vi "五子棋_電腦對戰V2.vi"() -> ()   [LabVIEW 2019, in "五子棋.lvlib"]
uses:
  Status.ctl
  SetPiece.ctl
  Piece.ctl
  <vilib>/numeric/Random Number (Range) U64.vi
  1e88ba00-7128-4acd-b617-a9aca016128f.vi
  <vilib>/numeric/sub_Random U32.vi
panel:
  out "Info":string
  out "狀態":string
  out "黑子":T1[][](array[typedef])
  out "白子":T2[][](array[typedef])
  out "Score":i32[][](array[numeric])
  # "五子棋電腦對戰版"
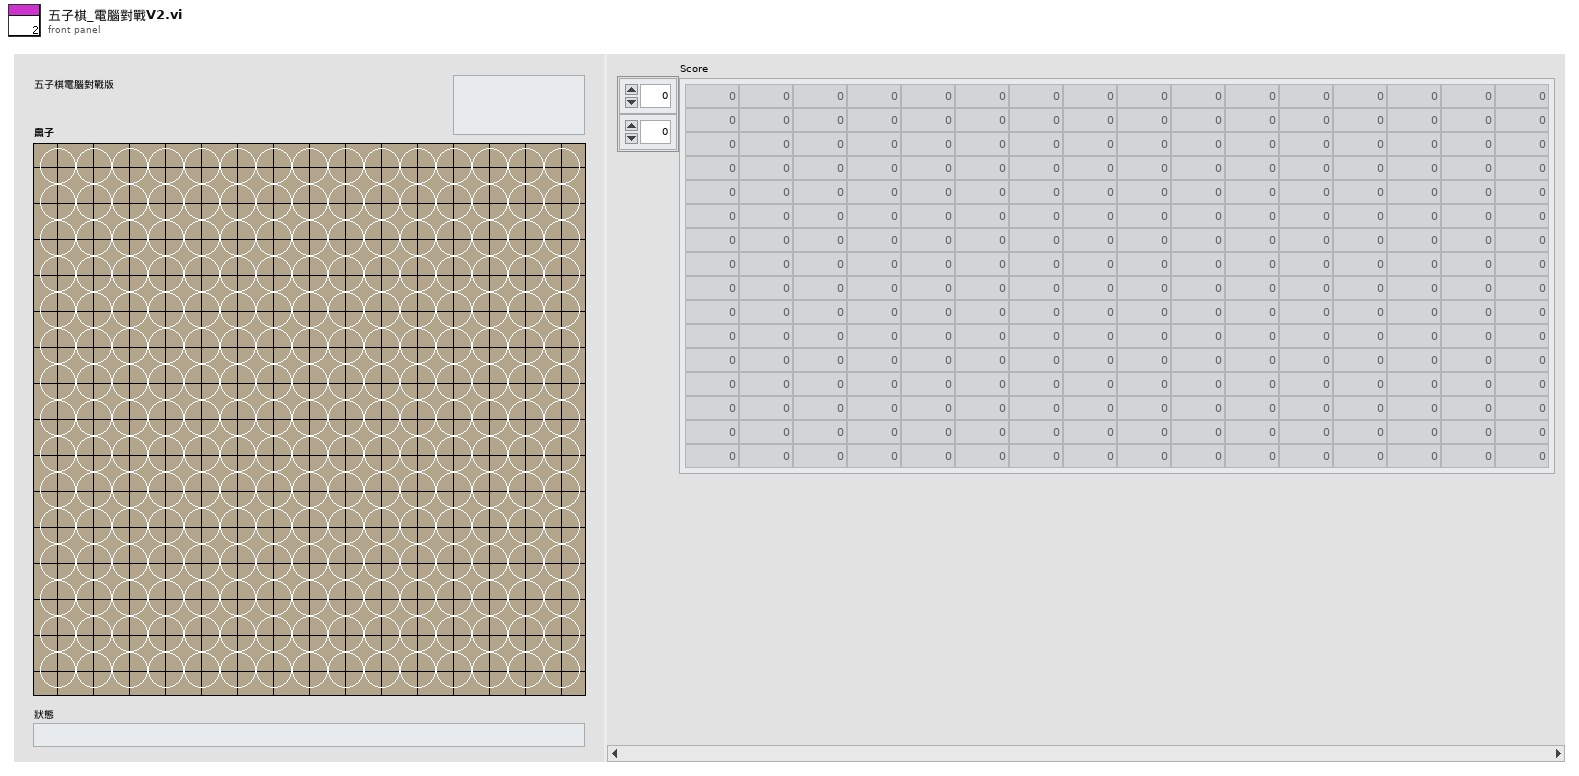
[diagram p1: front panel]
types:
  T1 = typedef "五子棋.lvlib/黑子.ctl" = bool
  T2 = typedef "五子棋.lvlib/白子.ctl" = bool
  T3 = typedef "五子棋.lvlib/Piece.ctl" = enum16{"None", "Black", "White"}
  T4 = typedef "五子棋.lvlib/SetPiece.ctl" = cluster{"Row":i32, "Col":i32}
  T5 = typedef "五子棋.lvlib/Status.ctl" = enum16{"Idle", "Initialize", "Set Piece", "Check Win", "Computer Play"}
  T6 = typedef "LVPositionTypeDef.ctl" = cluster{"Left":i32, "Top":i32}
  T7 = typedef "LVBoundsTypeDef.ctl" = cluster{"Width":u32, "Height":u32}
  T8 = cluster{"Number of Columns":u32, "Number of Rows":u32}
  T9 = typedef "LVPoint32TypeDef.ctl" = cluster{"Horizontal":i32, "Vertical":i32}
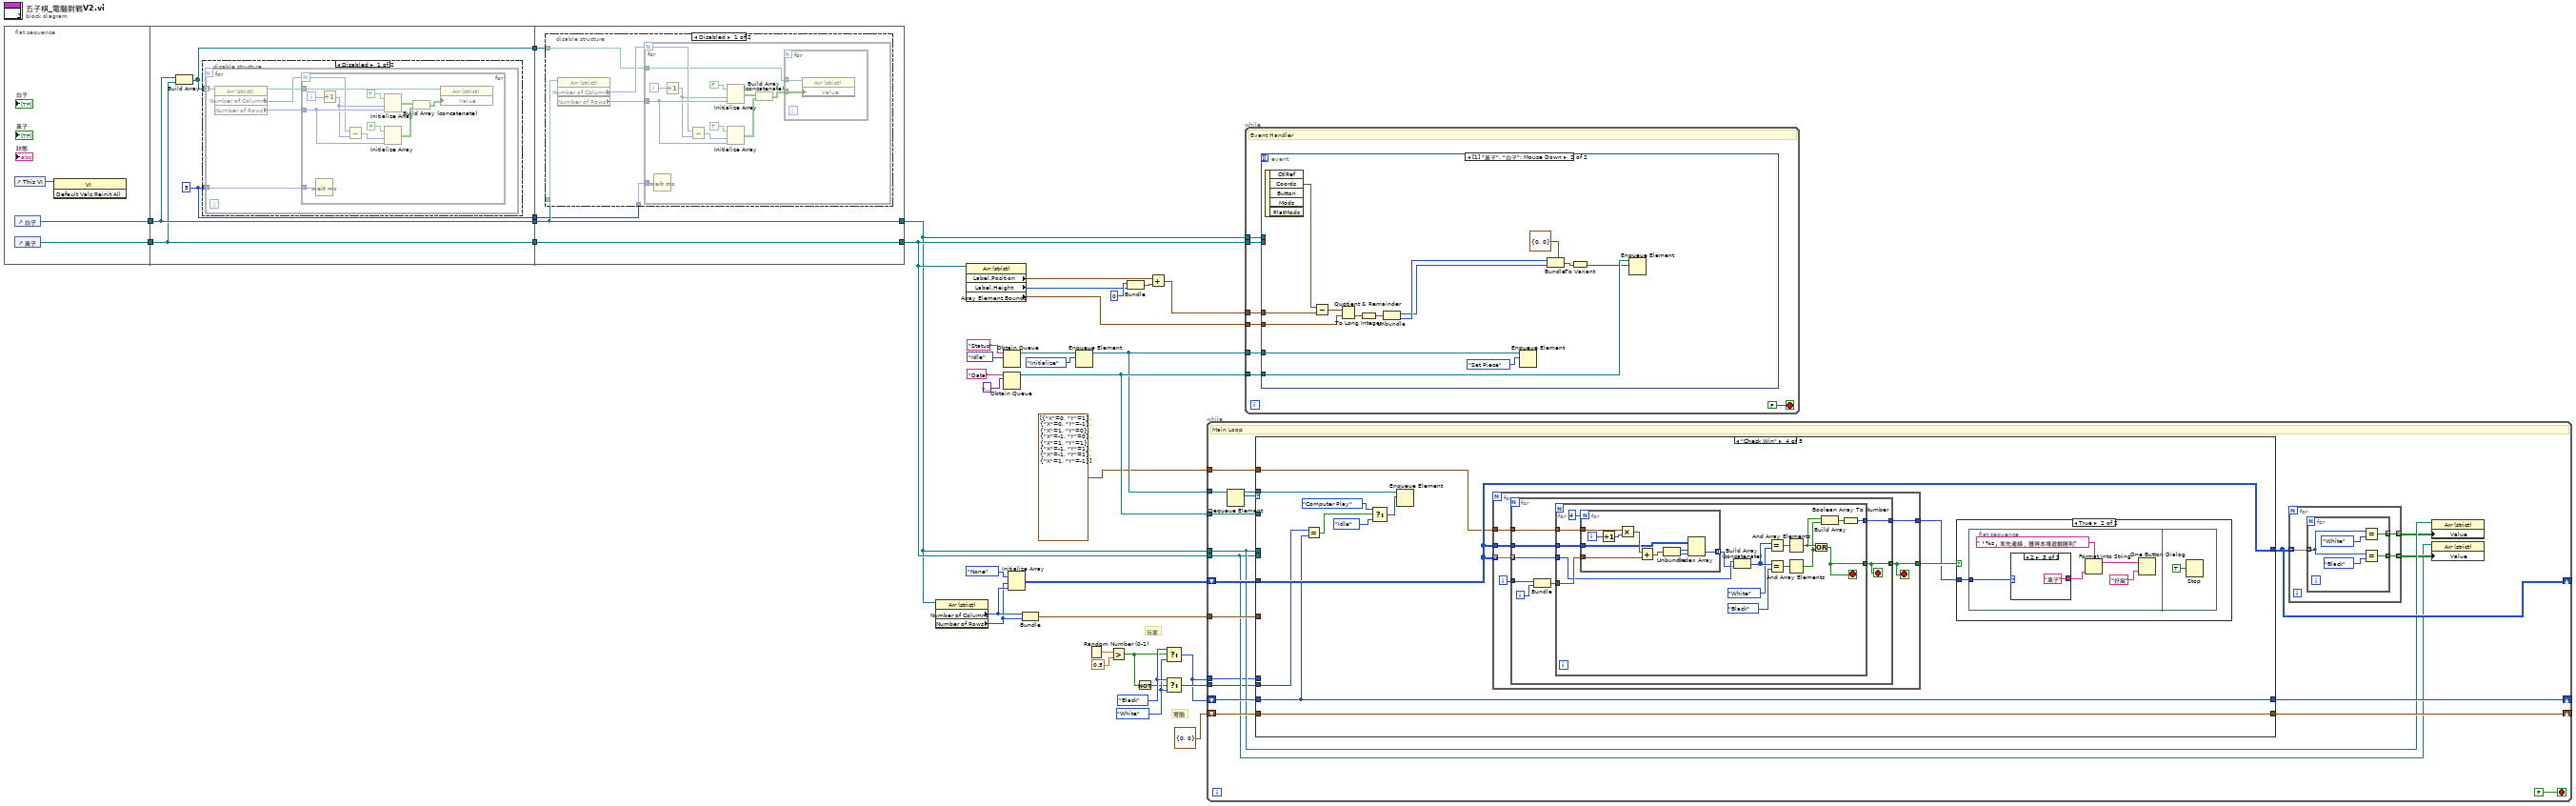
[diagram p0: block diagram]
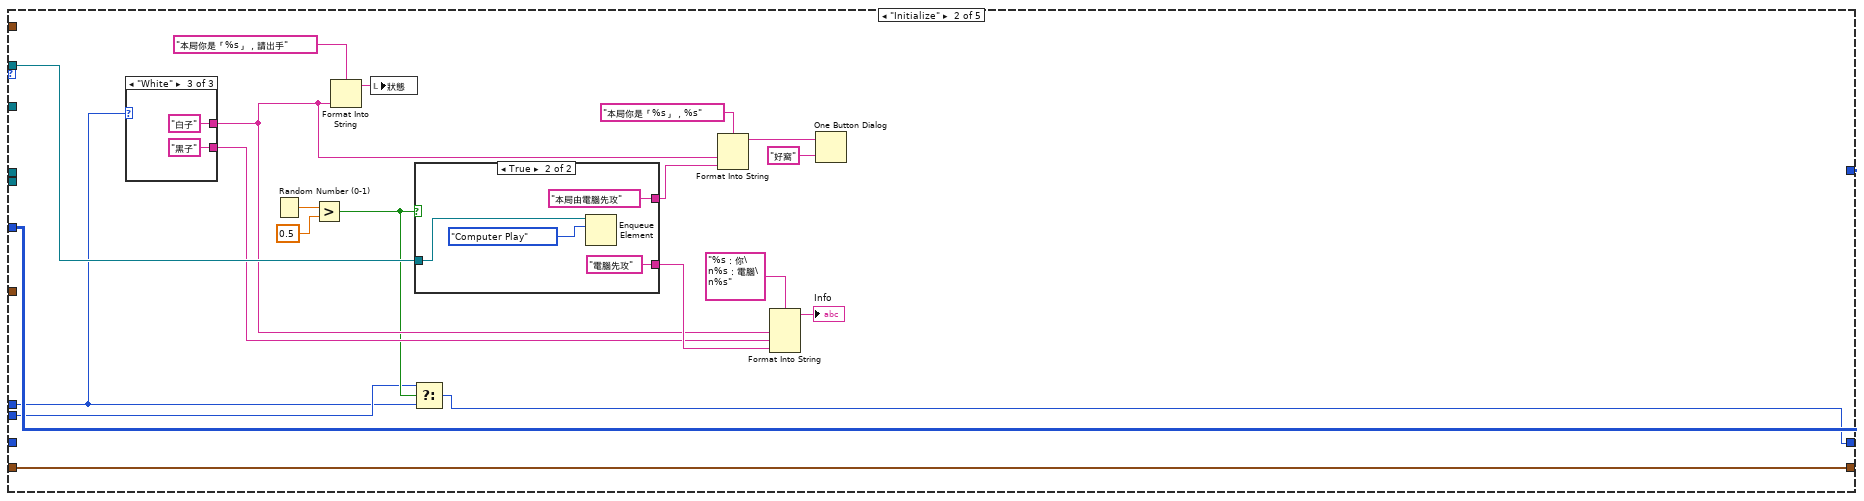
[diagram p5: hidden frame]
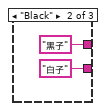
[diagram p7: hidden frame]
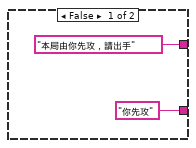
[diagram p8: hidden frame]
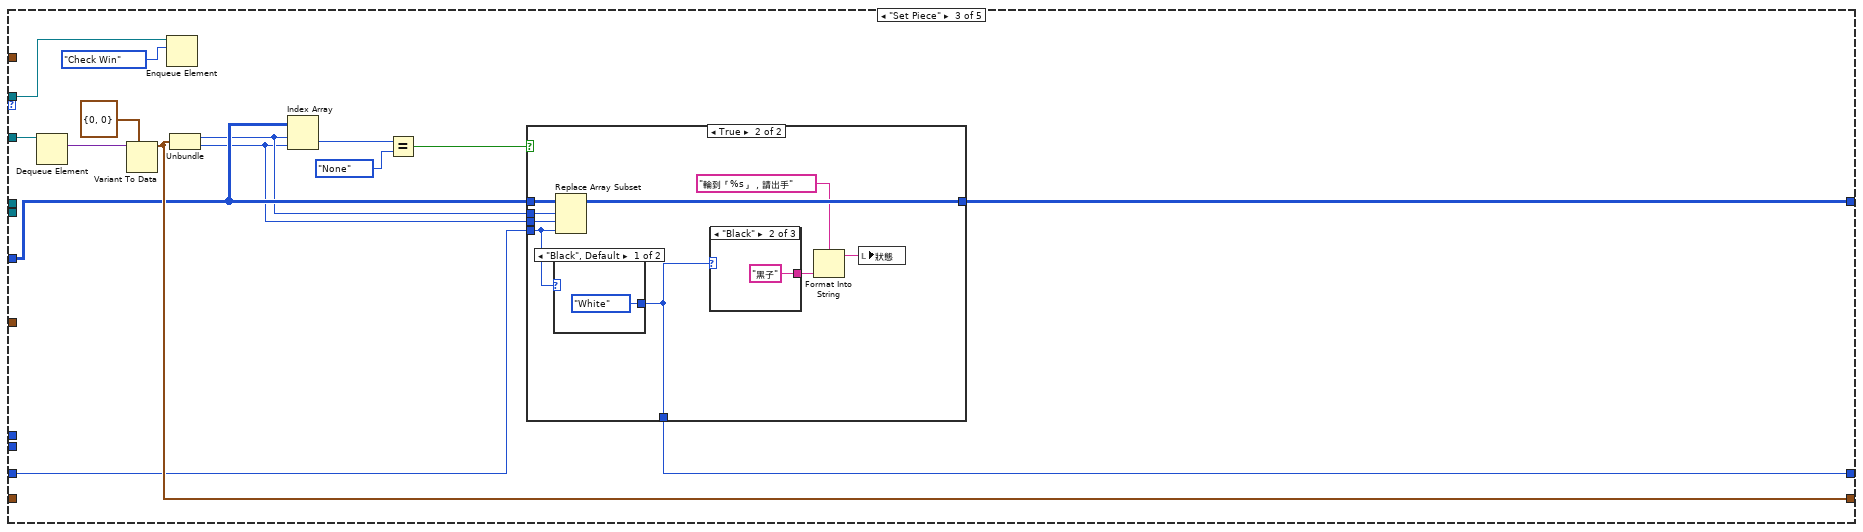
[diagram p9: hidden frame]
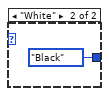
[diagram p11: hidden frame]
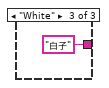
[diagram p13: hidden frame]
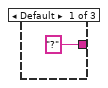
[diagram p15: hidden frame]
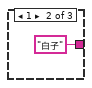
[diagram p16: hidden frame]
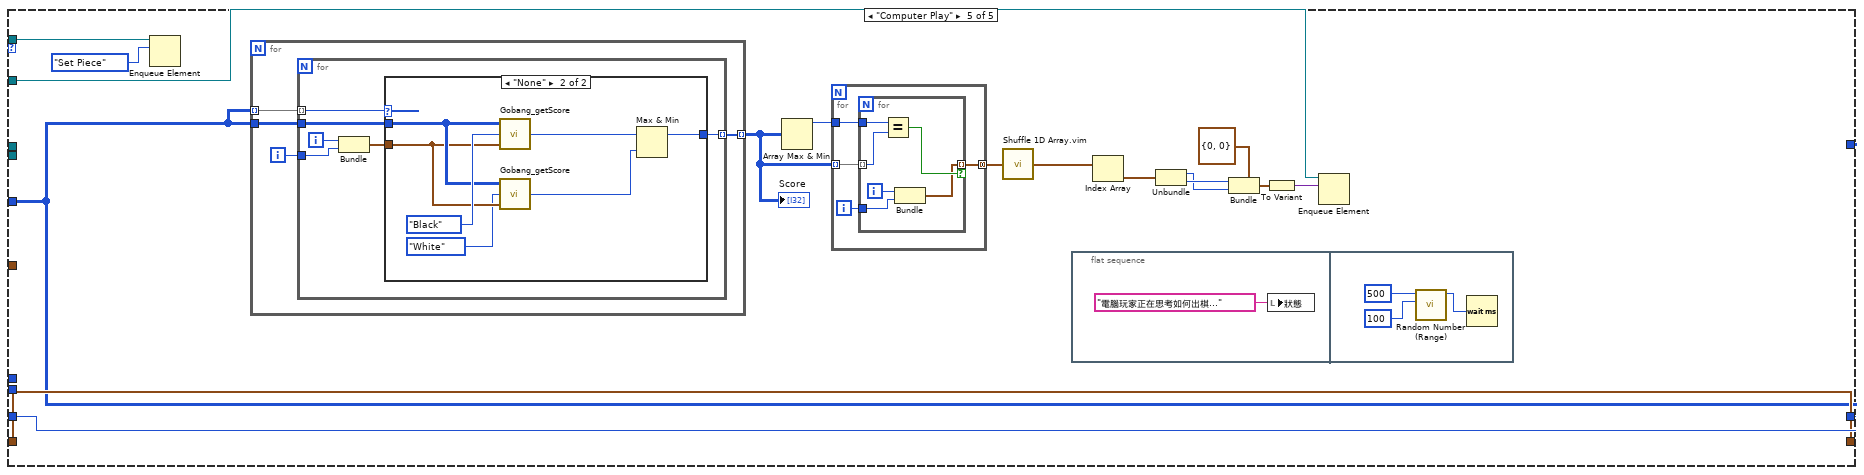
[diagram p17: hidden frame]
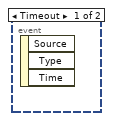
[diagram p19: hidden frame]
diagram:
  w7 = Piece."White" ("new element/subarray")
  w8 = Piece."Black" ("new element/subarray")
  # "電腦"
  # "玩家"
  n1 = flat-sequence {
    tunnel: [w39] -> w21
    tunnel: [w38] -> w20
    tunnel: w21 -> [w43]
    tunnel: w20 -> [w44]
    tunnel: [w43] -> w19
    tunnel: [w44] -> w18
    tunnel: [w42] -> w17
    tunnel: [w41] -> w13
    tunnel: [w66] -> w15
    tunnel: [w67] -> w32
    tunnel: w19 -> [w67]
    tunnel: w18 -> [w66]
    tunnel: w17 -> [w65]
    tunnel: w13 -> [w64]
    frame #0 {
      n2 = control-ref of="This VI"() -> (w40:refnum<vi>)
      n3 = control-ref of="白子"() -> (w38:refnum<vi>)
      n4 = control-ref of="黑子"() -> (w39:refnum<vi>)
      n5 = invoke class="VI" method="Default Vals.Reinit All"(reference=w40) -> ()  [unwired: 2 in, 3 out]
    }
    frame #1 {
      w41 = u32 5 ("milliseconds to wait")
      n6 = Build Array(w44, w43) -> (w42:refnum<vi>[])
      n7 = disable-structure shown="Disabled" {
        disable-tunnel: w42 -> [w46 _]
        disable-tunnel: w41 -> [w45 _]
        frame Disabled {
          n8 = for {
            tunnel: w46 -> [w51] mode=indexing
            tunnel: w45 -> [w47]
            n9 = property class="Arr (strict)"(reference=w51) -> (reference out=w48:refnum<vi>, "Number of Columns"=w50:u32, "Number of Rows"=w49:u32)  [unwired: 1 in, 1 out]
            n10 = for {
              N: w50 -> [w59]
              tunnel: w49 -> [w60]
              tunnel: w48 -> [w54]
              tunnel: w47 -> [w52]
              i -> [w62]
              n11 = Wait (ms)(milliseconds to wait=w52) -> ()  [unwired: 1 out]
              n12 = Increment(x=w62) -> (x+1=w58:i32)
              n13 = Subtract(x=w59, y=w58) -> (x-y=w57:i32)
              n14 = Initialize Array(TRUE, w58, w60) -> (w56:bool[][])
              n15 = Initialize Array(FALSE, w57, w60) -> (w55:bool[][])
              n16 = Build Array (concatenate)(w56, w55) -> (w53:bool[][])
              n17 = property class="Arr (strict)"(reference=w54, "Value"=w53) -> ()  [unwired: 1 in, 2 out]
            }
          }
        }
        frame Enabled {
        }
      }
    }
    frame #2 {
      n18 = disable-structure shown="Disabled" {
        disable-tunnel: w66 -> [w70 _]
        disable-tunnel: w65 -> [w69 _]
        disable-tunnel: w64 -> [w68 _]
        frame Disabled {
          n19 = property class="Arr (strict)"(reference=w70) -> ("Number of Columns"=w72:u32, "Number of Rows"=w71:u32)  [unwired: 1 in, 2 out]
          n20 = for {
            N: w72 -> [w80]
            tunnel: w71 -> [w81]
            tunnel: w69 -> [w74]
            tunnel: w68 -> [w73]
            i -> [w83]
            n21 = Wait (ms)(milliseconds to wait=w73) -> ()  [unwired: 1 out]
            n22 = Increment(x=w83) -> (x+1=w79:i32)
            n23 = Subtract(x=w80, y=w79) -> (x-y=w78:i32)
            n24 = Initialize Array(FALSE, w79, w81) -> (w77:bool[][])
            n25 = Initialize Array(TRUE, w78, w81) -> (w76:bool[][])
            n26 = Build Array (concatenate)(w77, w76) -> (w75:bool[][])
            n27 = for {
              tunnel: w74 -> [w86] mode=indexing
              tunnel: w75 -> [w85]
              n28 = property class="Arr (strict)"(reference=w86, "Value"=w85) -> ()  [unwired: 1 in, 2 out]
            }
          }
        }
        frame Enabled {
        }
      }
    }
  }
  n29 = property class="Arr (strict)"(reference=w15) -> ("Number of Columns"=w11:u32, "Number of Rows"=w10:u32)  [unwired: 1 in, 2 out]
  n30 = property class="Arr (strict)"(reference=w32) -> ("Label.Position"=w31:T6, "Label.Height"=w27:u32, "Array Element.Bounds"=w26:T7)  [unwired: 1 in, 2 out]
  n31 = Obtain Queue(name (unnamed)="Status", element data type=Status."Idle" ("Status")) -> (queue out=w23:refnum<queue>)  [unwired: 3 in, 2 out]
  n32 = Obtain Queue(name (unnamed)="Data", element data type=variant) -> (queue out=w33:refnum<queue>)  [unwired: 3 in, 2 out]
  n33 = Initialize Array(Piece."None", w10, w11) -> (w9:T3[][])
  n34 = Bundle("Number of Columns"=w11, "Number of Rows"=w10) -> (w3:T8)  [unwired: 1 in]
  n35 = Enqueue Element(queue=w23, element=Status."Initialize" ("Status")) -> (queue out=w14:refnum<queue>)  [unwired: 2 in, 2 out]
  n36 = Random Number (0-1)() -> (number: 0 to 1=w25:dbl)
  n37 = Greater?(x=w25, y=0.5) -> (0:w6:bool)
  n38 = Bundle(0, "Label.Height"=w27) -> (w30:cluster{i32, "Label.Height":u32})  [unwired: 1 in]
  n39 = Not(x=w6) -> (.not. x?=w5:bool)
  n40 = Add(x=w31, y=w30) -> (x+y=w29:cluster{i32, u32})
  n41 = Select(t=w8, s=w6, f=w7) -> (s? t:f=w1:T3)
  n42 = Select(t=w8, s=w5, f=w7) -> (s? t:f=w4:T3)
  n43 = while {
    tunnel: w14 -> [w104]
    tunnel: w33 -> [w100]
    tunnel: w32 -> [w90]
    tunnel: w15 -> [w93]
    shift-right: [w99] -> _
    shift-left: w1 -> [w98]
    shift-right: [w97] -> _
    shift-left: T4 {"Row"=0, "Col"=0} -> [w96]
    tunnel: w3 -> [w95]
    shift-right: [w105] -> _
    shift-left: w9 -> [w94]
    tunnel: w1 -> [w89]
    tunnel: w4 -> [w88]
    tunnel: cluster{"X":i32, "Y":i32}[] [{"X"=0, "Y"=1}, {"X"=0, "Y"=-1}, {"X"=1, "Y"=0}, {"X"=-1, "Y"=0}, {"X"=1, "Y"=1}, {"X"=-1, "Y"=1}, {"X"=-1, "Y"=1}, {"X"=1, "Y"=-1}] -> [w87]
    stop <- FALSE stop-if-true
    # "Main Loop"
    n44 = Dequeue Element(queue=w104) -> (queue out=w101:refnum<queue>, element=w103:T5)  [unwired: 2 in, 2 out]
    n45 = case shown="\"Check Win\"" w103 {
      tunnel: w90 -> [_ _ _ _ _]
      tunnel: w93 -> [_ _ _ _ _]
      tunnel: w101 -> [_ w125 w152 w180 w246]
      tunnel: w100 -> [_ _ w150 _ w240]
      tunnel: [w108 w109 w139 w171 w245] -> w99
      tunnel: w98 -> [w108 _ w146 w171 w245]
      tunnel: [w107 w126 w148 w174 w243] -> w97
      tunnel: w96 -> [w107 w126 _ w174 w243]
      tunnel: w95 -> [_ _ _ _ _]
      tunnel: w94 -> [w106 w115 w145 w173 w242]
      tunnel: [w106 w115 w147 w173 w242] -> w105
      tunnel: w89 -> [_ w110 _ _ _]
      tunnel: w88 -> [_ w111 _ w170 _]
      tunnel: w87 -> [_ _ _ w169 _]
      frame "Idle", Default {
      }
      frame "Initialize" {
        n46 = case shown="\"White\"" w110 {
          tunnel: [_ "黑子" "白子"] -> w114
          tunnel: [_ "白子" "黑子"] -> w113
          frame Default {
          }
          frame "Black" {
          }
          frame "White" {
          }
        }
        n47 = Random Number (0-1)() -> (number: 0 to 1=w123:dbl)
        n48 = Greater?(x=w123, y=0.5) -> (0:w112:bool)
        n49 = Format Into String(format string="本局你是「%s」，請出手", w114) -> (resulting string=w127:string)  [unwired: 2 in, 1 out]
        n50 = local write "狀態"(w127) -> ()
        n51 = Select(t=w111, s=w112, f=w110) -> (s? t:f=w109:T3)
        n52 = case shown="True" w112 {
          tunnel: w125 -> [_ w136]
          tunnel: ["本局由你先攻，請出手" ("format string") "本局由電腦先攻" ("format string")] -> w121
          tunnel: ["你先攻" ("format string") "電腦先攻" ("format string")] -> w117
          frame False {
          }
          frame True {
            n53 = Enqueue Element(queue=w136, element=Status."Computer Play" ("Status")) -> ()  [unwired: 2 in, 3 out]
          }
        }
        n54 = Format Into String(format string="本局你是「%s」，%s", w114, w121) -> (resulting string=w120:string)  [unwired: 2 in, 1 out]
        n55 = Format Into String(format string="%s：你\n%s：電腦\n%s", w114, w113, w117) -> (resulting string=→"Info":string)  [unwired: 2 in, 1 out]
        n56 = One Button Dialog(message=w120, button name ("OK")="好窩") -> ()  [unwired: 1 out]
      }
      frame "Set Piece" {
        n57 = Dequeue Element(queue=w150) -> (element=w149:variant)  [unwired: 2 in, 3 out]
        n58 = Variant To Data(type=T4 {"Row"=0, "Col"=0}, Variant=w149) -> (data=w148:T4)  [unwired: 1 in, 1 out]
        n59 = Enqueue Element(queue=w152, element=Status."Check Win") -> ()  [unwired: 2 in, 3 out]
        n60 = Unbundle(w148) -> ("Row"=w144:i32, "Col"=w143:i32)
        n61 = Index Array(array=w145, index (row)=w144, index (col)=w143) -> (element=w142:T3)
        n62 = Equal?(x=w142, y=Piece."None") -> (x = y?=w140:bool)
        n63 = case shown="True" w140 {
          tunnel: [w155 w164] -> w147
          tunnel: w146 -> [w154 w158]
          tunnel: w145 -> [w155 w163]
          tunnel: w144 -> [_ w162]
          tunnel: w143 -> [_ w161]
          tunnel: [w154 w156] -> w139
          frame False {
          }
          frame True {
            n64 = case shown="\"Black\", Default" w158 {
              tunnel: [Piece."White" ("new element/subarray") Piece."Black" ("new element/subarray")] -> w156
              frame "Black", Default {
              }
              frame "White" {
              }
            }
            n65 = Replace Array Subset(array=w163, new element=w158, index (row)=w162, index (col)=w161) -> (w164:T3[][])
            n66 = case shown="\"Black\"" w156 {
              tunnel: [_ "黑子" "白子"] -> w160
              frame Default {
              }
              frame "Black" {
              }
              frame "White" {
              }
            }
            n67 = Format Into String(format string="輪到「%s」，請出手", w160) -> (resulting string=w159:string)  [unwired: 2 in, 1 out]
            n68 = local write "狀態"(w159) -> ()
          }
        }
      }
      frame "Check Win" {
        n69 = Equal?(x=w170, y=w171) -> (x = y?=w178:bool)
        n70 = Select(t=Status."Computer Play" ("element"), s=w178, f=Status."Idle" ("element")) -> (s? t:f=w177:T5)
        n71 = Enqueue Element(queue=w180, element=w177) -> ()  [unwired: 2 in, 3 out]
        n72 = for {
          tunnel: [w186] -> w179
          tunnel: w173 -> [w184] mode=indexing
          tunnel: w173 -> [w183]
          tunnel: [w182] -> w172
          tunnel: w169 -> [w181]
          i -> [w185]
          stop <- w186 stop-if-true
          n73 = for {
            tunnel: [w194] -> w186
            tunnel: w185 -> [w193]
            tunnel: w184 -> [w190] mode=indexing
            tunnel: w183 -> [w189]
            tunnel: [w188] -> w182
            tunnel: w181 -> [w187]
            i -> [w192]
            stop <- w194 stop-if-true
            n74 = Bundle(w193, w192) -> (w191:cluster{i32, i32})  [unwired: 1 in]
            n75 = for {
              tunnel: [w200] -> w194
              tunnel: w191 -> [w209]
              tunnel: w190 -> [w207]
              tunnel: w189 -> [w208]
              tunnel: [w196] -> w188
              tunnel: w187 -> [w195] mode=indexing
              stop <- w200 stop-if-true
              n76 = for {
                N: 4 -> [_]
                tunnel: w209 -> [w218]
                tunnel: w208 -> [w213]
                tunnel: [w212] -> w206 mode=indexing
                tunnel: w195 -> [w211]
                i -> [w217]
                n77 = Increment(x=w217) -> (x+1=w216:i32)
                n78 = Multiply(x=w211, y=w216) -> (x*y=w215:cluster{"X":i32, "Y":i32})
                n79 = Add(x=w215, y=w218) -> (x+y=w214:cluster{i32, i32})
                n80 = Unbundle(w214) -> (w220:i32, w219:i32)
                n81 = Index Array(array=w213, index (row)=w220, index (col)=w219) -> (element=w212:T3)
              }
              n82 = Build Array (concatenate)(w207, w206) -> (w202:T3[])
              n83 = Equal?(x=w202, y=Piece."White") -> (x = y?=w203:bool[])
              n84 = Equal?(x=w202, y=Piece."Black") -> (x = y?=w204:bool[])
              n85 = And Array Elements(Boolean array=w203) -> (logical AND=w199:bool)
              n86 = And Array Elements(Boolean array=w204) -> (logical AND=w198:bool)
              n87 = Or(x=w199, y=w198) -> (x .or. y?=w200:bool)
              n88 = Build Array(w199, w198) -> (w197:bool[])
              n89 = Boolean Array To Number(Boolean array=w197) -> (number=w196:u32)
            }
          }
        }
        n90 = case shown="True" w179 {
          tunnel: w172 -> [_ w221]
          frame False {
          }
          frame True {
            n91 = flat-sequence {
              tunnel: w221 -> [w222]
              frame #0 {
                n92 = case shown="2" w222 {
                  tunnel: ["?" "白子" "黑子"] -> w225
                  frame Default {
                  }
                  frame 1 {
                  }
                  frame 2 {
                  }
                }
                n93 = Format Into String(format string="「%s」率先連線，獲得本場遊戲勝利", w225) -> (resulting string=w224:string)  [unwired: 2 in, 1 out]
                n94 = One Button Dialog(message=w224, button name ("OK")="好窩") -> ()  [unwired: 1 out]
              }
              frame #1 {
                n95 = Stop(stop? (T)=TRUE) -> ()
              }
            }
          }
        }
      }
      frame "Computer Play" {
        n96 = Enqueue Element(queue=w246, element=Status."Set Piece") -> ()  [unwired: 2 in, 3 out]
        n97 = for {
          tunnel: w242 -> [w264]
          tunnel: w242 -> [w263] mode=indexing
          tunnel: [w262] -> w231 mode=indexing
          i -> [w261]
          n98 = for {
            tunnel: w264 -> [w270]
            tunnel: w263 -> [w265] mode=indexing
            tunnel: [w268] -> w262 mode=indexing
            tunnel: w261 -> [w266]
            i -> [w267]
            n99 = Bundle(w267, w266) -> (w269:cluster{i32, i32})  [unwired: 1 in]
            n100 = case shown="\"None\"" w265 {
              tunnel: w270 -> [_ w276]
              tunnel: w269 -> [_ w275]
              tunnel: [_ w271] -> w268
              frame Default {
              }
              frame "None" {
                n101 = call "Gobang_getScore.vi"("Position"=w275, "Color"=Piece."Black", "Topo"=w276) -> ("Score"=w273:i32)
                n102 = call "Gobang_getScore.vi"("Position"=w275, "Color"=Piece."White", "Topo"=w276) -> ("Score"=w272:i32)
                n103 = Max & Min(x=w273, y=w272) -> (max(x,y)=w271:i32)  [unwired: 1 out]
              }
            }
          }
        }
        "Score" <- w231
        n104 = Array Max & Min(array=w231) -> (max value=w239:i32)  [unwired: 3 out]
        n105 = for {
          tunnel: w231 -> [w253] mode=indexing
          tunnel: w239 -> [w254]
          tunnel: [w251] -> w238 mode=concatenating
          i -> [w252]
          n106 = for {
            tunnel: w254 -> [w260]
            tunnel: w253 -> [w259] mode=indexing
            tunnel: [w255] -> w251 mode=indexing if=w258
            tunnel: w252 -> [w256]
            i -> [w257]
            n107 = Equal?(x=w260, y=w259) -> (x = y?=w258:bool)
            n108 = Bundle(w257, w256) -> (w255:cluster{i32, i32})  [unwired: 1 in]
          }
        }
        n109 = call "Shuffle 1D Array.vim"("array"=w238) -> ("shuffled array"=w237:cluster{i32, i32}[])  [unwired: 4 in]
        n110 = flat-sequence {
          frame #0 {
            n111 = local write "狀態"("電腦玩家正在思考如何出棋..." ("狀態")) -> ()
          }
          frame #1 {
            n112 = call-poly <vilib>:"Random Number (Range).vi"("lower bound (0)"=u64 100, "upper bound (100)"=u64 500 ("lower bound (0)")) -> ("number"=w248:u64)  [unwired: 9 in]
            n113 = Wait (ms)(milliseconds to wait=w248) -> ()  [unwired: 1 out]
          }
        }
        n114 = Index Array(array=w237) -> (element=w236:cluster{i32, i32})  [unwired: 1 in]
        n115 = Unbundle(w236) -> (w233:i32, w234:i32)
        n116 = Bundle(cluster=T4 {"Row"=0, "Col"=0}, "Row"=w234, "Col"=w233) -> (w232:T4)
        n117 = To Variant(anything=w232) -> (Variant=w241:variant)
        n118 = Enqueue Element(queue=w240, element=w241) -> ()  [unwired: 2 in, 3 out]
      }
    }
    n119 = for {
      tunnel: w105 -> [w280] mode=indexing
      tunnel: [w279] -> w92 mode=indexing
      tunnel: [w278] -> w91 mode=indexing
      n120 = for {
        tunnel: w280 -> [w283] mode=indexing
        tunnel: [w282] -> w279 mode=indexing
        tunnel: [w281] -> w278 mode=indexing
        n121 = Equal?(x=w283, y=Piece."White") -> (x = y?=w282:bool)
        n122 = Equal?(x=w283, y=Piece."Black") -> (x = y?=w281:bool)
      }
    }
    n123 = property class="Arr (strict)"(reference=w93, "Value"=w92) -> ()  [unwired: 1 in, 2 out]
    n124 = property class="Arr (strict)"(reference=w90, "Value"=w91) -> ()  [unwired: 1 in, 2 out]
  }
  n125 = while {
    tunnel: w32 -> [w291]
    tunnel: w15 -> [w290]
    tunnel: w26 -> [w289]
    tunnel: w14 -> [w288]
    tunnel: w33 -> [w287]
    tunnel: w29 -> [w286]
    stop <- FALSE stop-if-true
    # "Event Handler"
    n126 = event shown="[1] \"黑子\", \"白子\": Mouse Down" {
      selector: _ -> [_ _]
      dyn-events: _ -> [_ _]
      timeout: _ -> [_ _]
      tunnel: w291 -> [_ _]
      tunnel: w290 -> [_ _]
      tunnel: w289 -> [_ w298]
      tunnel: w288 -> [_ w303]
      tunnel: w287 -> [_ w302]
      tunnel: w286 -> [_ w300]
      event Timeout {
        n127 = event-data() -> ()  [unwired: 1 in, 3 out]
      }
      event "黑子", "白子": Mouse Down {
        n128 = event-data() -> ("Coords"=w301:T9)  [unwired: 1 in, 4 out]
        n129 = Subtract(x=w301, y=w300) -> (x-y=w299:cluster{i32, u32})
        n130 = Quotient & Remainder(x=w299, y=w298) -> (floor(x/y)=w297:T7)  [unwired: 1 out]
        n131 = To Long Integer(number=w297) -> (32bit integer=w306:cluster{"Width":i32, "Height":i32})
        n132 = Unbundle(w306) -> ("Width"=w304:i32, "Height"=w305:i32)
        n133 = Enqueue Element(queue=w303, element=Status."Set Piece") -> ()  [unwired: 2 in, 3 out]
        n134 = Bundle(cluster=T4 {"Row"=0, "Col"=0}, "Row"=w305, "Col"=w304) -> (w294:T4)
        n135 = To Variant(anything=w294) -> (Variant=w293:variant)
        n136 = Enqueue Element(queue=w302, element=w293) -> ()  [unwired: 2 in, 3 out]
      }
    }
  }
